vi "convert 24bit to 1bit.vi"(9 "colors":T2={"color diff"=FALSE, "On color"=0, "Off color"=16777215}, 11 "image data":T1) -> (1 "middle color":u32(colorbox), 2 "1-bit pixmap":bool[][](array[boolean]))   [LabVIEW 2009]
uses:
  <vilib>/picture/picture.llb/imagedata.ctl
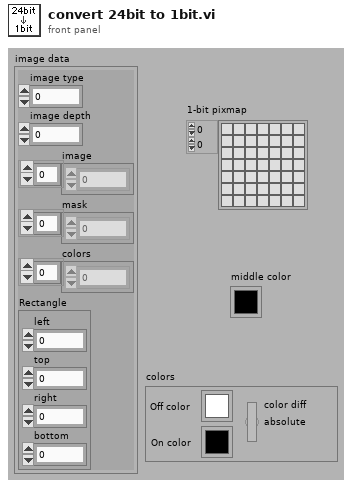
[diagram p1: front panel]
types:
  T1 = typedef "imagedata.ctl" = cluster{"image type":i32, "image depth":i32, "image":u8[], "mask":u8[], "colors":u32[], "Rectangle":cluster{"left":i16, "top":i16, "right":i16, "bottom":i16}}
  T2 = cluster{"color diff":bool, "On color":u32, "Off color":u32}
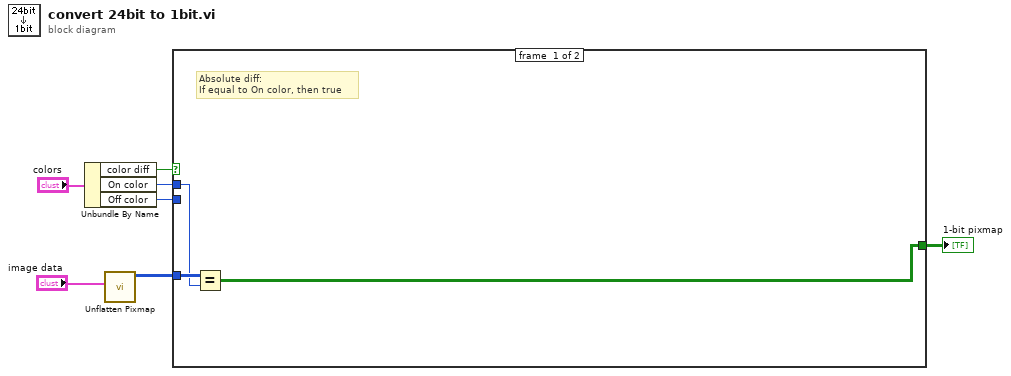
[diagram p0: block diagram]
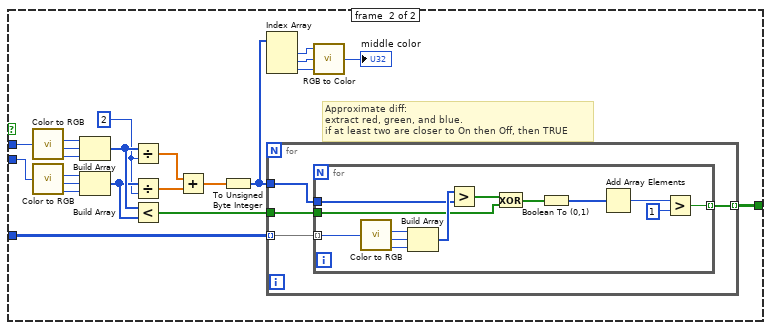
[diagram p2: hidden frame]
diagram:
  n1 = Unbundle By Name("colors") -> ("color diff"=w3:bool, "On color"=w5:u32, "Off color"=w4:u32)
  n2 = call <vilib>:"Unflatten Pixmap.vi"("image data"="image data") -> ("24-bit pixmap"=w2:u32[][])  [unwired: 4 in, 6 out]
  n3 = case shown="True" w3 {
    tunnel: w5 -> [w9 w32]
    tunnel: w4 -> [_ w31]
    tunnel: w2 -> [w10 w23]
    tunnel: [w8 w16] -> w1
    frame #0 {
      # "Absolute diff:\nIf equal to On color, then true"
      n4 = Equal?(x=w10, y=w9) -> (x = y?=w8:bool[][])
    }
    frame #1 {
      w18 = 2
      # "Approximate diff:\nextract red, green, and blue.\nif at least two are closer to On then Off, then TRUE"
      n5 = call <vilib>:"Color to RGB.vi"("Color"=w32) -> ("R"=w25:u8, "G"=w26:u8, "B"=w27:u8)  [unwired: 1 out]
      n6 = call <vilib>:"Color to RGB.vi"("Color"=w31) -> ("R"=w28:u8, "G"=w30:u8, "B"=w29:u8)  [unwired: 1 out]
      n7 = Build Array(w25, w26, w27) -> (w22:u8[])
      n8 = Build Array(w28, w30, w29) -> (w21:u8[])
      n9 = Divide(x=w22, y=w18) -> (x/y=w20:dbl[])
      n10 = Divide(x=w21, y=w18) -> (x/y=w19:dbl[])
      n11 = Less?(x=w22, y=w21) -> (x < y?=w17:bool[])
      n12 = Add(x=w20, y=w19) -> (x+y=w24:dbl[])
      n13 = To Unsigned Byte Integer(number=w24) -> (unsigned 8bit integer=w15:u8[])
      n14 = Index Array(array=w15) -> (element #1=w14:u8, element #2=w13:u8, element #3=w12:u8)  [unwired: 3 in]
      n15 = for {
        tunnel: w23 -> [w36] mode=indexing
        tunnel: w15 -> [w35]
        tunnel: w17 -> [w34]
        tunnel: [w33] -> w16 mode=indexing
        n16 = for {
          tunnel: w36 -> [w49] mode=indexing
          tunnel: w35 -> [w44]
          tunnel: w34 -> [w42]
          tunnel: [w37] -> w33 mode=indexing
          n17 = call <vilib>:"Color to RGB.vi"("Color"=w49) -> ("R"=w48:u8, "G"=w47:u8, "B"=w46:u8)  [unwired: 1 out]
          n18 = Build Array(w48, w47, w46) -> (w45:u8[])
          n19 = Greater?(x=w45, y=w44) -> (0:w43:bool[])
          n20 = Exclusive Or(1:w42, 2:w43) -> (0:w41:bool[])
          n21 = Boolean To (0,1)(Boolean=w41) -> (0, 1=w40:i16[])
          n22 = Add Array Elements(numeric array=w40) -> (sum=w39:i16)
          n23 = Greater?(x=w39, y=i16 1) -> (0:w37:bool)
        }
      }
      n24 = call <vilib>:"RGB to Color.vi"("B"=w12, "G"=w13, "R"=w14) -> ("Color"=→"middle color":u32)
    }
  }
  "1-bit pixmap" <- w1
